vi "FF_FindClosestPtFromTraj.vi"(10 "AnkleInGCS":dbl[](array[numeric]), 11 "AnkleTraj":T1[](array[typedef])) -> (0 "ClosestPt":dbl[](array[numeric]), 1 "DistanceToClosestPt":dbl, 2 "NormalVectorToClosestPt":dbl[](array[numeric]), 3 "TangentVectorAtClosestPt":dbl[](array[numeric]), 5 "IndexOfClosePt":i32)   [LabVIEW 2016, in "ForceField.lvclass"]
uses:
  ForceField.lvclass
  TypeDef/AnkleTrajPt.ctl
  <vilib>/Analysis/baseanly.llb/Real Dot Product.vi
  <vilib>/Analysis/_algsub.llb/Real Vector Norm.vi
  <vilib>/Analysis/NI_AALBase.lvlib
  <vilib>/Analysis/NI_AALPro.lvlib
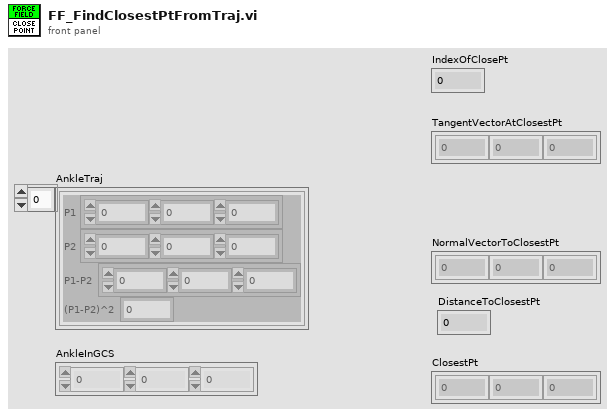
[diagram p1: front panel]
types:
  T1 = typedef "ForceField.lvclass/AnkleTrajPt.ctl" = cluster{"P1":dbl[], "P2":dbl[], "P1-P2":dbl[], "(P1-P2)^2":dbl}
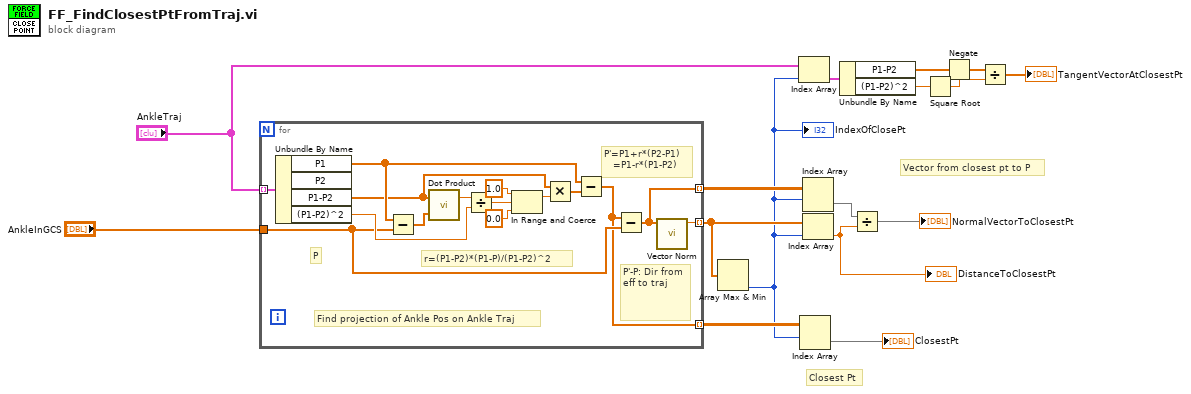
[diagram p0: block diagram]
diagram:
  # "Vector from closest pt to P"
  # "Closest Pt"
  n1 = for {
    tunnel: "AnkleTraj" -> [w31] mode=indexing
    tunnel: "AnkleInGCS" -> [w18]
    tunnel: [w22] -> w3 mode=indexing
    tunnel: [w21] -> w11 mode=indexing
    tunnel: [w17] -> w15 mode=indexing
    # "P"
    # "P'-P: Dir from eff to traj"
    # "r=(P1-P2)*(P1-P)/(P1-P2)^2"
    # "P'=P1+r*(P2-P1)\n   =P1-r*(P1-P2)"
    # "Find projection of Ankle Pos on Ankle Traj"
    n2 = Unbundle By Name(w31) -> ("P1"=w23:dbl[], "P1-P2"=w20:dbl[], "(P1-P2)^2"=w19:dbl)  [unwired: 1 out]
    n3 = Subtract(x=w23, y=w18) -> (x-y=w30:dbl[])
    n4 = call-poly <vilib>:"Dot Product.vi"("Y Vector"=w30, "X Vector"=w20) -> ("X * Y"=w29:dbl)  [unwired: 1 out]
    n5 = Divide(x=w29, y=w19) -> (x/y=w28:dbl)
    n6 = In Range and Coerce(upper limit=1.0, x=w28, lower limit=0.0) -> (coerced(x)=w25:dbl)  [unwired: 1 out]
    n7 = Multiply(x=w20, y=w25) -> (x*y=w24:dbl[])
    n8 = Subtract(x=w23, y=w24) -> (x-y=w17:dbl[])
    n9 = Subtract(x=w17, y=w18) -> (x-y=w21:dbl[])
    n10 = call-poly <vilib>:"Vector Norm.vi"("Input Vector"=w21) -> ("norm"=w22:dbl)  [unwired: 9 in, 1 out]
  }
  n11 = Array Max & Min(array=w3) -> (min index (indices)=w2:i32)  [unwired: 3 out]
  "IndexOfClosePt" <- w2
  n12 = Index Array(array="AnkleTraj", index=w2) -> (element=w5:T1)
  n13 = Index Array(array=w15, index (row)=w2) -> (element=→"ClosestPt":dbl[])  [unwired: 1 in]
  n14 = Index Array(array=w11, index (row)=w2) -> (element=w12:dbl[])  [unwired: 1 in]
  n15 = Index Array(array=w3, index=w2) -> (element=w14:dbl)
  "DistanceToClosestPt" <- w14
  n16 = Unbundle By Name(w5) -> ("P1-P2"=w9:dbl[], "(P1-P2)^2"=w10:dbl)
  n17 = Divide(x=w12, y=w14) -> (x/y=→"NormalVectorToClosestPt":dbl[])
  n18 = Square Root(x=w10) -> (sqrt(x)=w8:dbl)
  n19 = Negate(x=w9) -> (-x=w7:dbl[])
  n20 = Divide(x=w7, y=w8) -> (x/y=→"TangentVectorAtClosestPt":dbl[])
